vi "Get Report String.vi"(8 "error in (no error)":errorcluster, 11 "TestStand Result Handler In":refnum<class "TestStand Result Handler.lvclass">) -> (0 "error out":errorcluster, 2 "Report Text":string)   [LabVIEW 2020, in "Astemes_CSVReportPlugin.lvlib" / "TestStand Result Handler.lvclass"]
uses:
  TestStand Result Handler.lvclass
  TestStand Result Handler.lvclass/TestStand Result Handler.ctl
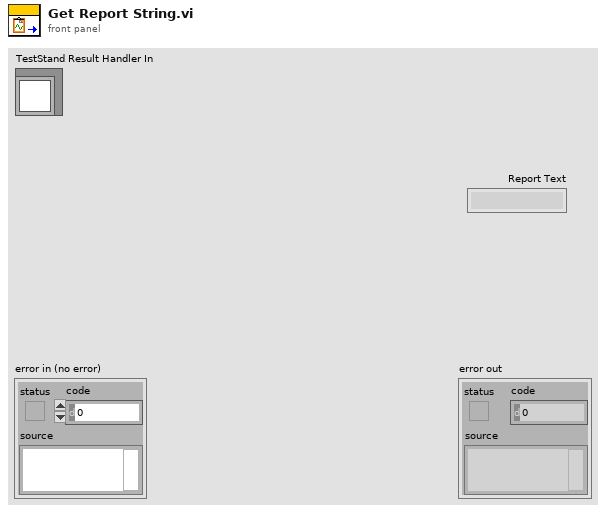
[diagram p1: front panel]
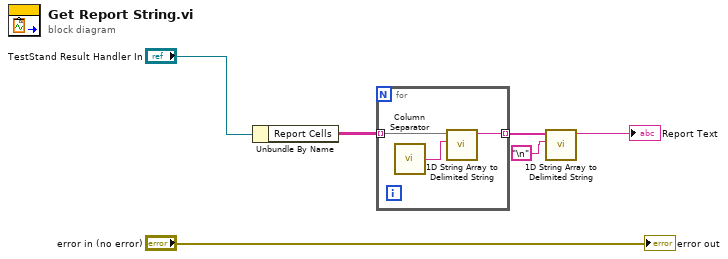
[diagram p0: block diagram]
diagram:
  n1 = Unbundle By Name("TestStand Result Handler In") -> ("Report Cells"=w4:string[][])
  n2 = for {
    tunnel: w4 -> [w9] mode=indexing
    tunnel: [w8] -> w3 mode=indexing
    n3 = call "Column Separator.vi"() -> ("delimiter"=w7:string)
    n4 = call <vilib>:"1D String Array to Delimited String.vi"("delimiter"=w7, "string array"=w9) -> ("delimited string"=w8:string)  [unwired: 9 in]
  }
  n5 = call <vilib>:"1D String Array to Delimited String.vi"("delimiter"="\n", "string array"=w3) -> ("delimited string"=→"Report Text":string)  [unwired: 9 in]
  "error out" <- "error in (no error)"
